vi "EX 3-2 RGB LED.vi"() -> ()   [LabVIEW 2011, in "LabVIEW Interface for Arduino.lvlib"]
doc: "An example that uses the Arduino's PWM pins to control an RGB LED."
uses:
  <vilib>/LabVIEW Interface for Arduino/LabVIEW Interface for Arduino.lvlib
panel:
  out "Color":u32(colorbox)
  in  "Blue":u8(slide) scale=0.0..255.0
  in  "Green":u8(slide) scale=0.0..255.0
  in  "Stop":bool
  in  "Red":u8(slide) scale=0.0..255.0
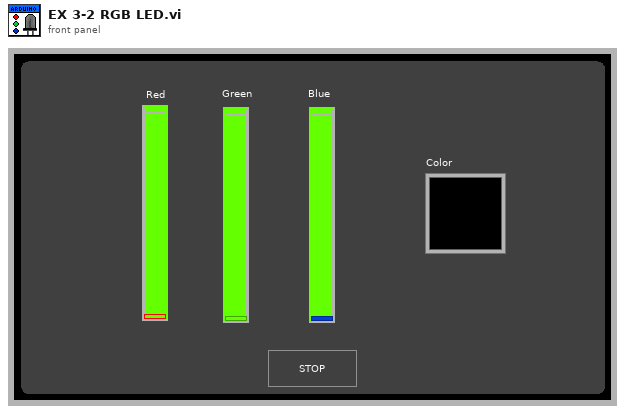
[diagram p1: front panel]
types:
  T1 = typedef "LabVIEW Interface for Arduino.lvlib/Arduino Resource.ctl" = cluster{"VISA resource":refnum<visa-resource-name>, "Board Type":T2, "Connection Type":enum8{"USB / Serial"}, "Bytes Per Packet (15)":u8}
  T2 = typedef "LabVIEW Interface for Arduino.lvlib/Board Type.ctl" = enum16{"Uno", "Dimuelanove w/Atmega 328", "Mega 2560"}
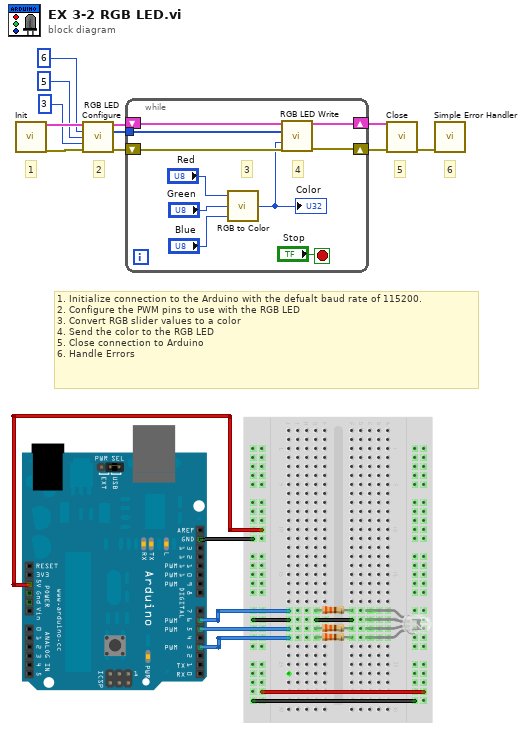
[diagram p0: block diagram]
diagram:
  # "6"
  # "5"
  # "2"
  # "1"
  # "1. Initialize connection to the Arduino with the defualt baud rate of 115200.\n2. Configure the PWM pins to use with the RGB LED\n3. Convert RGB slider values to a color\n4. Send the color to the RGB LED\n5. Close connection to Arduino\n6. Handle Errors"
  n1 = call <vilib>:"Init.vi"() -> ("Arduino Resource"=w9:T1, "error out"=w10:errorcluster)  [unwired: 18 in]
  n2 = call <vilib>:"RGB LED Configure.vi"("Arduino Resource"=w9, "Red Pin"=u8 6, "Green Pin"=u8 5, "Blue Pin"=u8 3, "error in"=w10) -> ("Arduino Resource"=w8:T1, "RGB LED Pins"=w1:u8[], "error out"=w7:errorcluster)  [unwired: 8 in]
  n3 = while {
    shift-right: [w21] -> w2
    shift-left: w8 -> [w13]
    shift-right: [w20] -> w11
    shift-left: w7 -> [w19]
    tunnel: w1 -> [w12]
    stop <- "Stop" stop-if-true
    # "4"
    # "3"
    n4 = call <vilib>:"RGB to Color.vi"("B"="Blue", "G"="Green", "R"="Red") -> ("Color"=w16:u32)
    "Color" <- w16
    n5 = call <vilib>:"RGB LED Write.vi"("Arduino Resource"=w13, "RGB LED Pins"=w12, "Color"=w16, "error in"=w19) -> ("Arduino Resource"=w21:T1, "error out"=w20:errorcluster)  [unwired: 9 in, 1 out]
  }
  n6 = call <vilib>:"Close.vi"("Arduino Resource"=w2, "error in"=w11) -> ("error out"=w6:errorcluster)  [unwired: 13 in]
  n7 = call <vilib>:"Simple Error Handler.vi"("error in (no error)"=w6) -> ()  [unwired: 4 in, 5 out]
